vi "TestExec.Result, Config, Read Station ID Info and Generate Vars.vi"(11 "Config Dir":path) -> (3 "Vars":string[][](array[string]))   [LabVIEW 2019]
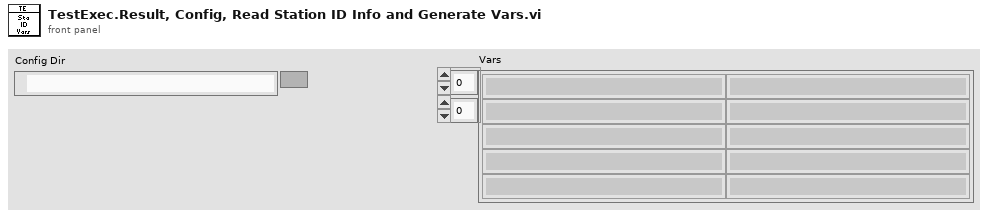
[diagram p1: front panel]
types:
  T1 = typedef "TestResult.Station Info.ctl" = cluster{"Name":string, "PN":string, "SN":string, "Rev":string, "PC Name":string, "Location":string, "HW_Config":cluster{"HW_Item":T2[]}, "SW_Config":cluster{"SW_Item":T3[]}}
  T2 = typedef "TestResult.HW Item.ctl" = cluster{"Name":string, "MFG":string, "PN":string, "SN":string, "SW/FW":string, "Note":string, "Cal_ID":string, "Cal_Type":string, "Cal_Due_Date":timestamp, "Cal_Status":string}
  T3 = typedef "TestResult.SW Item.ctl" = cluster{"Name":string, "PN":string, "Version":string, "Note":string}
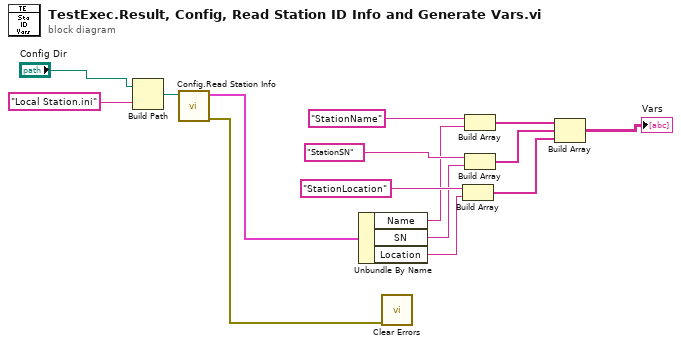
[diagram p0: block diagram]
diagram:
  n1 = Build Path(base path="Config Dir", name or relative path="Local Station.ini") -> (appended path=w6:path)
  n2 = call "Config.Read Station Info.vi"("Local Station Config File"=w6) -> ("error out"=w1:errorcluster, "Station"=w5:T1)  [unwired: 7 in, 2 out]
  n3 = Unbundle By Name(w5) -> ("Name"=w12:string, "SN"=w11:string, "Location"=w10:string)
  n4 = call <vilib>:"Clear Errors.vi"("error in (no error)"=w1) -> ()  [unwired: 5 in, 2 out]
  n5 = Build Array("StationLocation", w10) -> (w7:string[])
  n6 = Build Array("StationName", w12) -> (w9:string[])
  n7 = Build Array("StationSN", w11) -> (w8:string[])
  n8 = Build Array(w9, w8, w7) -> (→"Vars":string[][])
